vi "Private Read.vi"(8 "error in":errorcluster, 11 "Megger cluster in":T1={"Read data"={"Firmware version"="", "Model number"="", "Serial number"=0, "Ramp rate"=0.0, "Test Voltage"=0.0, "Test duration"=0.0, "Test stop watch"=0.0, "measured Current (nA)"=0.0, "calculated Resistance"=0.0, "Test Mode"=enum."Insulation resistance (IR)", "Test status"=enum."Waiting to start test"}, "Connected?"=FALSE, "Device status array"=[]}) -> (0 "error out":errorcluster, 2 "Serial read":string, 3 "Megger cluster out":T1={"Read data"={"Firmware version"="", "Model number"="", "Serial number"=0, "Ramp rate"=0.0, "Test Voltage"=0.0, "Test duration"=0.0, "Test stop watch"=0.0, "measured Current (nA)"=0.0, "calculated Resistance"=0.0, "Test Mode"=enum."Insulation resistance (IR)", "Test status"=enum."Waiting to start test"}, "Connected?"=FALSE, "Device status array"=[]})   [LabVIEW 2014]
uses:
  Controls/Megger cluster.ctl
  Controls/Global Megger.vi
  <vilib>/regexp/Match Regular Expression.xnode
  Stopwatch/Stop watch/Stop watch.lvlib
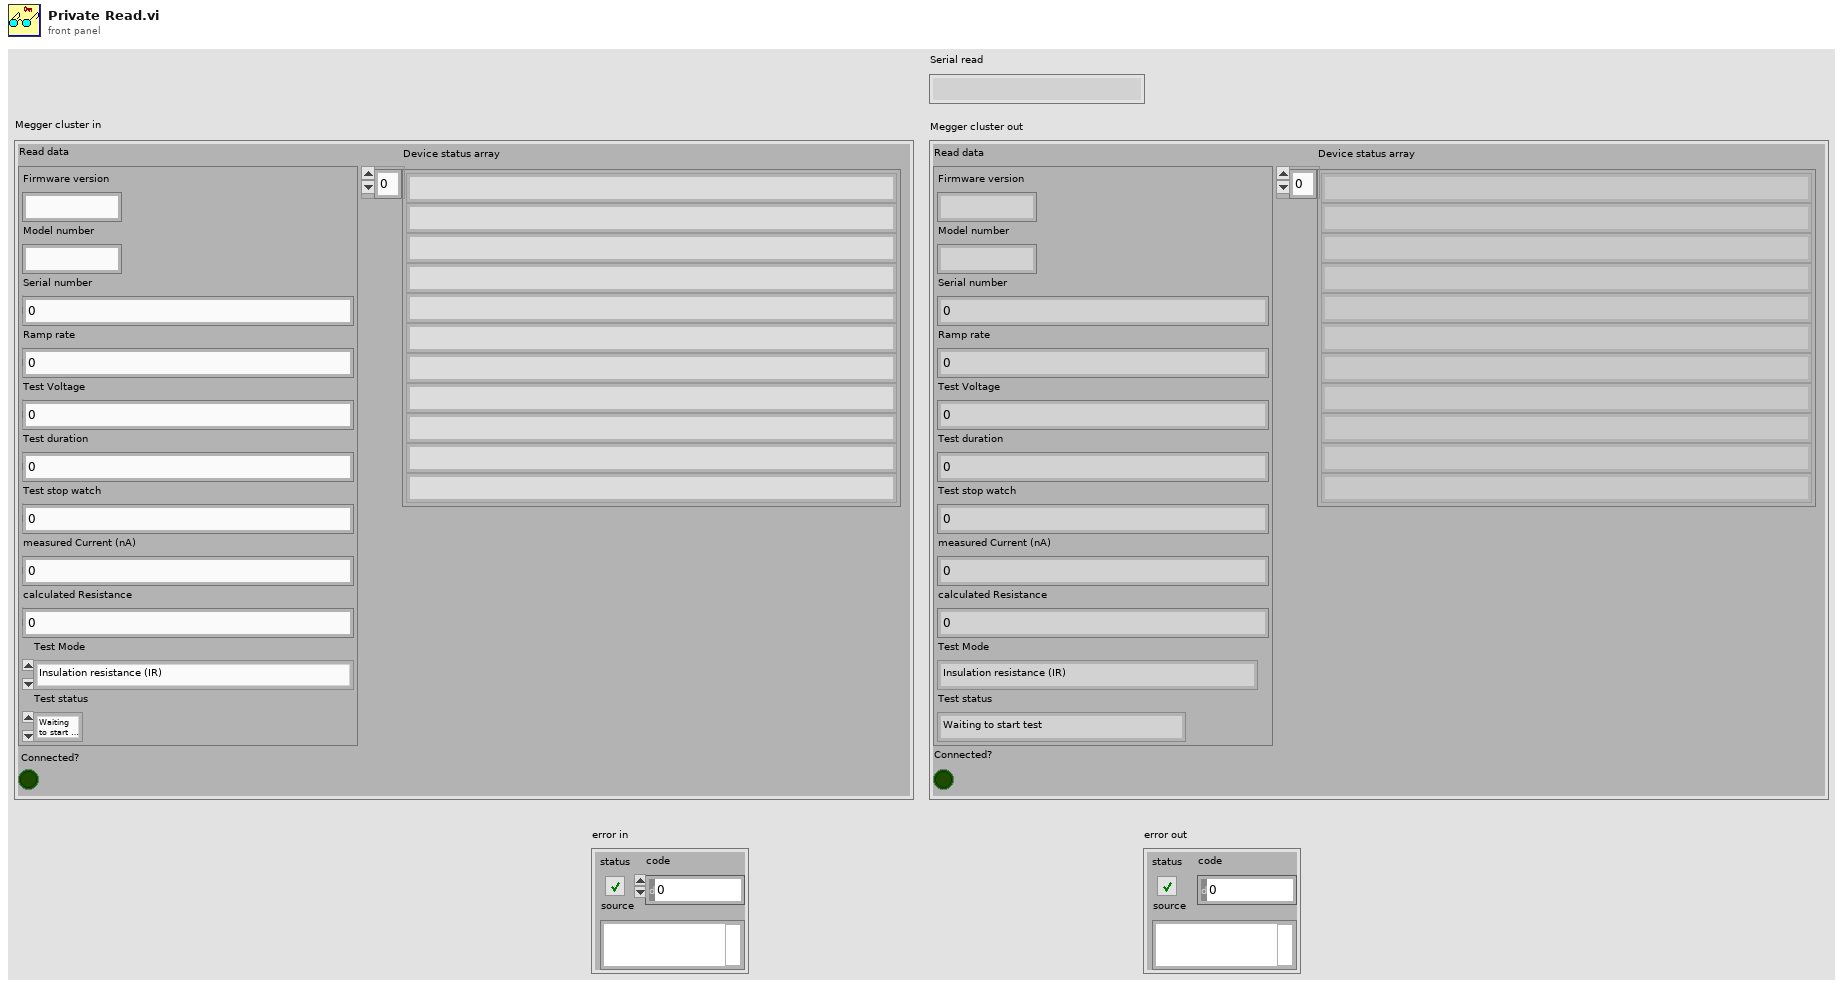
[diagram p1: front panel]
types:
  T1 = typedef "Megger cluster.ctl" = cluster{"Read data":cluster{"Firmware version":string, "Model number":string, "Serial number":i32, "Ramp rate":dbl, "Test Voltage":dbl, "Test duration":sgl, "Test stop watch":sgl, "measured Current (nA)":dbl, "calculated Resistance":dbl, "Test Mode":enum16{"N/A", "Insulation resistance (IR)", "Timed Insulation resistance (IR(t))", "Diaelectric Absorption Ratio (DAR)", "Polarisation Index (PI)", "Diaelectric Dishcharge (DD)", "Step voltage (SV)", "Ramp test (Ramp)"}, "Test status":enum16{"Waiting to start test", "Unable to start test", "Test progressing normally", "Performing post test measurements", "Test has ended normally", "Test has been aborted"}}, "Connected?":bool, "Device status array":string[]}
  T2 = enum16{"N/A", "Insulation resistance (IR)", "Timed Insulation resistance (IR(t))", "Diaelectric Absorption Ratio (DAR)", "Polarisation Index (PI)", "Diaelectric Dishcharge (DD)", "Step voltage (SV)", "Ramp test (Ramp)"}
  T3 = enum16{"Waiting to start test", "Unable to start test", "Test progressing normally", "Performing post test measurements", "Test has ended normally", "Test has been aborted"}
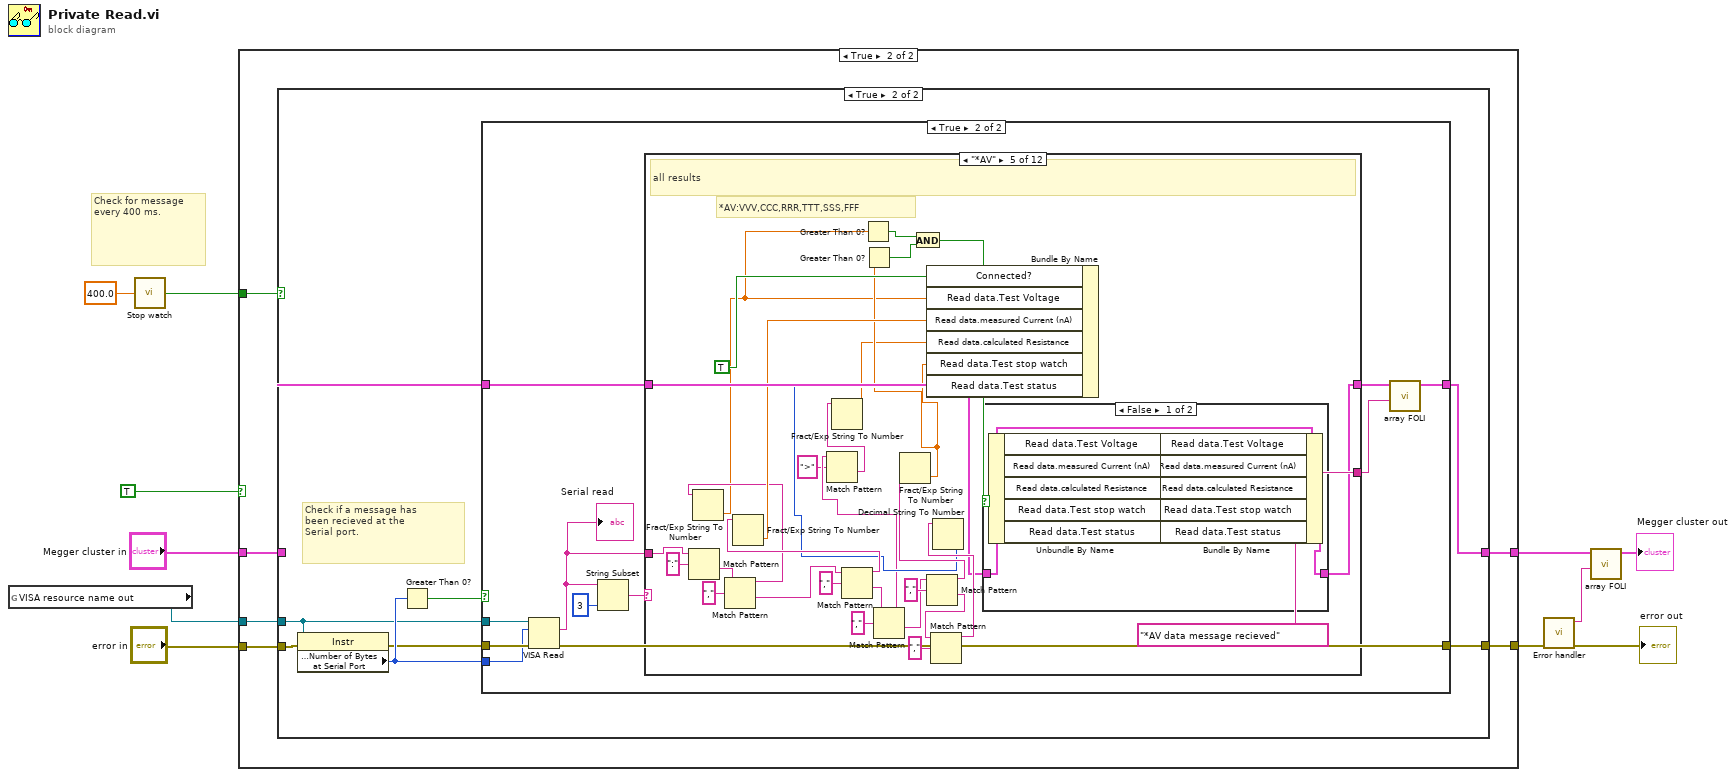
[diagram p0: block diagram]
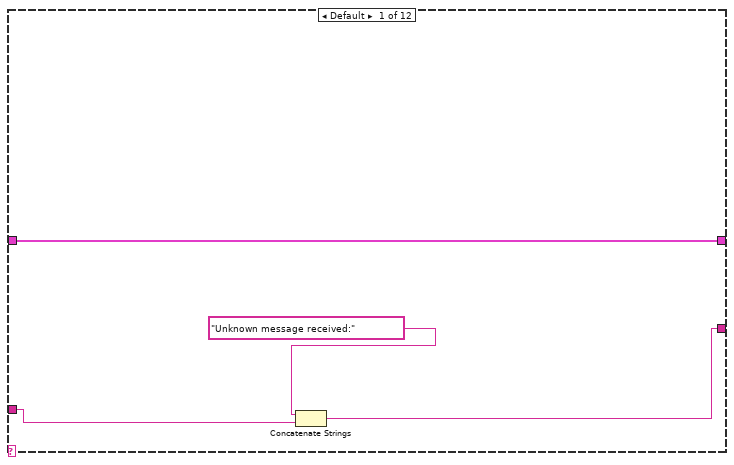
[diagram p5: hidden frame]
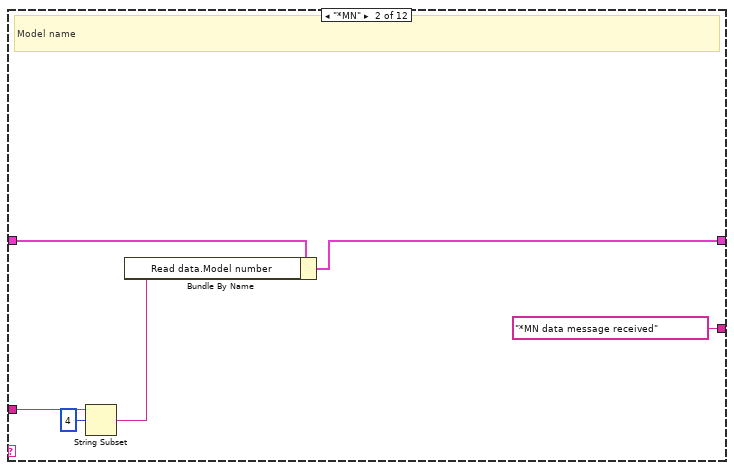
[diagram p6: hidden frame]
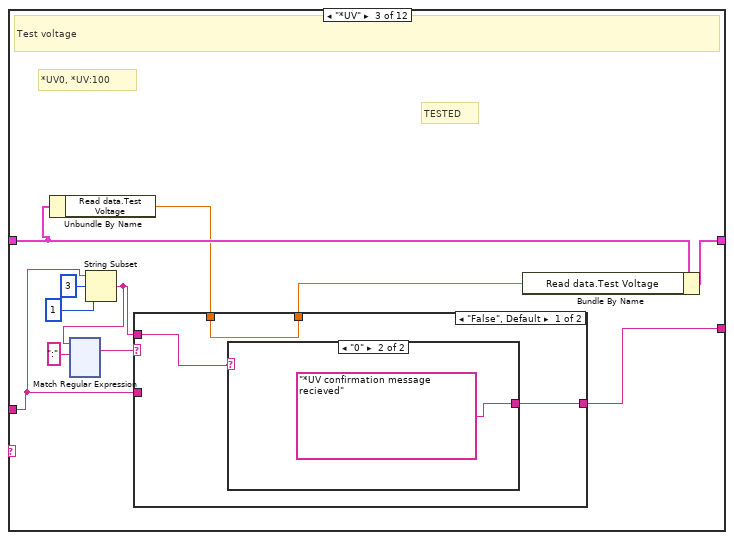
[diagram p7: hidden frame]
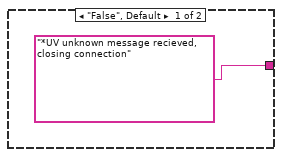
[diagram p8: hidden frame]
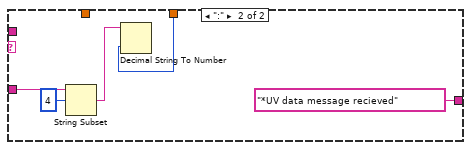
[diagram p9: hidden frame]
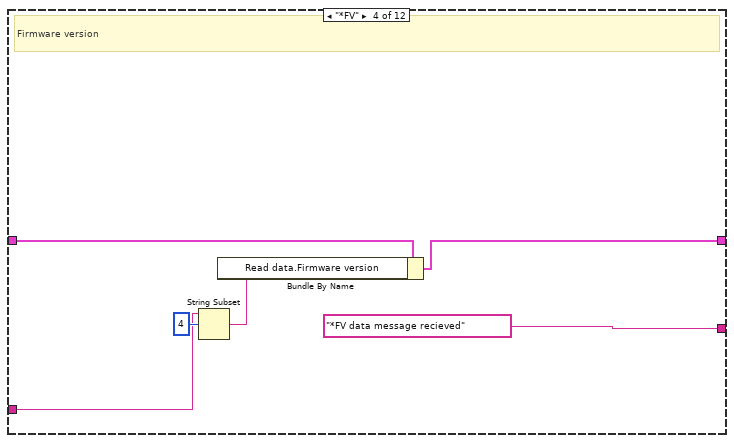
[diagram p10: hidden frame]
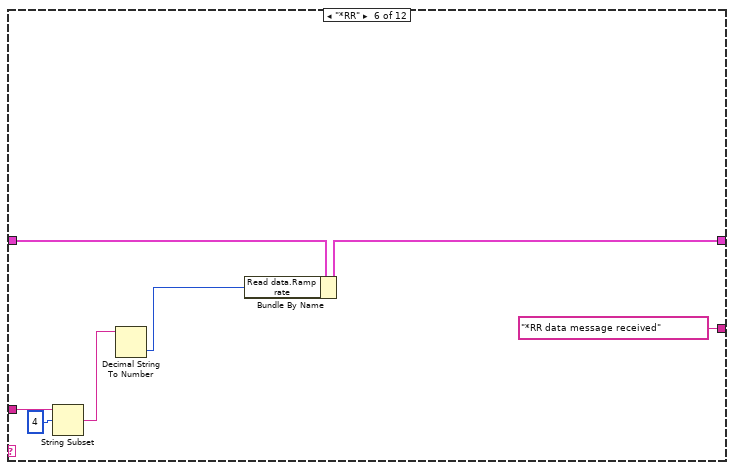
[diagram p12: hidden frame]
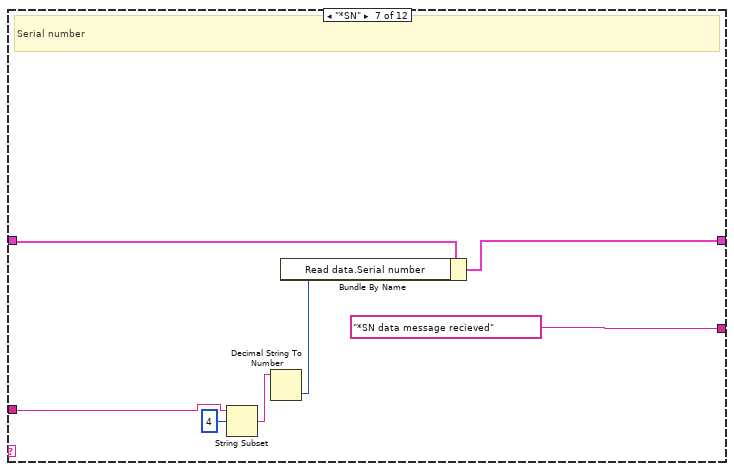
[diagram p13: hidden frame]
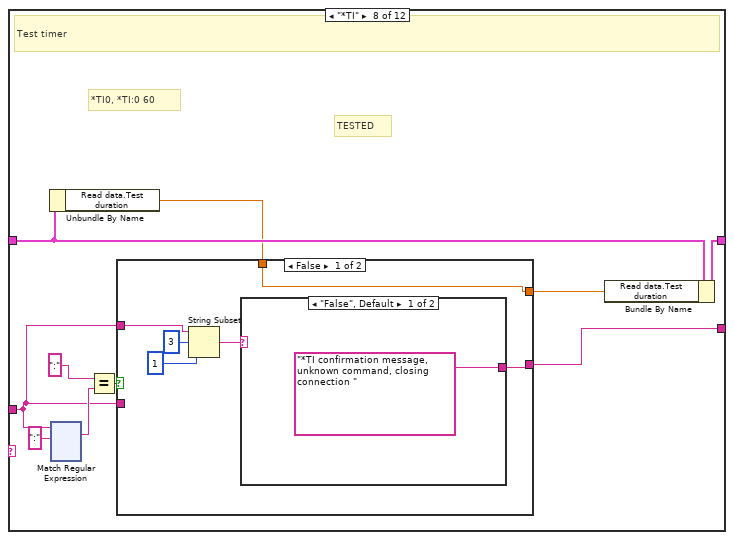
[diagram p14: hidden frame]
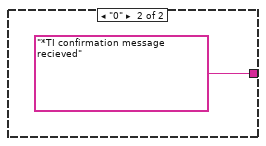
[diagram p15: hidden frame]
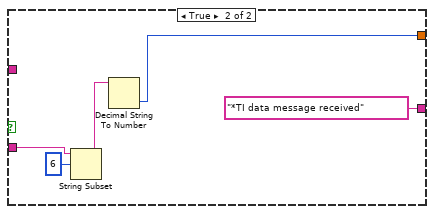
[diagram p16: hidden frame]
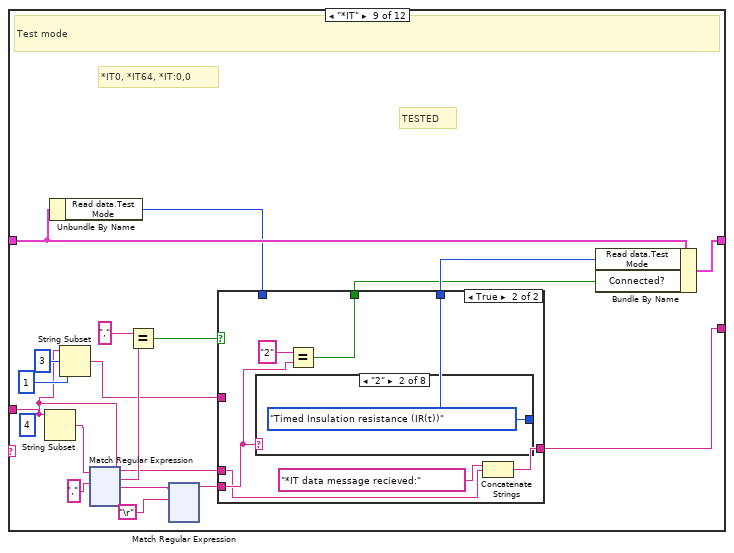
[diagram p17: hidden frame]
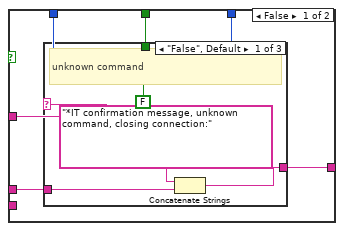
[diagram p18: hidden frame]
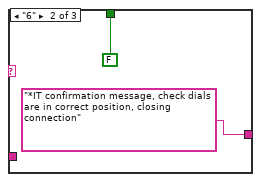
[diagram p19: hidden frame]
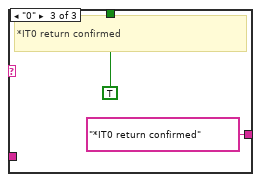
[diagram p20: hidden frame]
diagram:
  # "Check for message \nevery 400 ms."
  n1 = global read "Global Megger.vi" "VISA resource name out"() -> (w3:refnum<visa-resource-name>)
  n2 = call "Stop watch.vi"("Time to wait, mS"=400.0) -> ("Timer up"=w2:bool)  [unwired: 13 in, 1 out]
  n3 = case shown="True" TRUE {
    tunnel: [w13 w19] -> w8
    tunnel: "Megger cluster in" -> [w12 w18]
    tunnel: [w12 w17] -> w7
    tunnel: "error in" -> [w13 w16]
    tunnel: w2 -> [_ w15]
    tunnel: w3 -> [_ w14]
    frame False {
    }
    frame True {
      n4 = case shown="True" w15 {
        tunnel: [w21 w29] -> w19
        tunnel: w18 -> [w20 w28]
        tunnel: [w20 w27] -> w17
        tunnel: w16 -> [w21 w23]
        tunnel: w14 -> [_ w22]
        frame False {
        }
        frame True {
          # "Check if a message has \nbeen recieved at the\nSerial port."
          n5 = property class="Instr"(reference=w22, error in=w23) -> (error out=w24:errorcluster, "Serial Settings:Number of Bytes at Serial Port"=w25:u32)  [unwired: 1 out]
          n6 = Greater Than 0?(x=w25) -> (x > 0?=w26:bool)
          n7 = case shown="True" w26 {
            tunnel: [w31 w42] -> w29
            tunnel: w22 -> [_ w41]
            tunnel: w24 -> [w31 w40]
            tunnel: w25 -> [_ w39]
            tunnel: w28 -> [w30 w37]
            tunnel: [w30 w32] -> w27
            frame False {
            }
            frame True {
              n8 = VISA Read(VISA resource name=w41, byte count=w39, error in (no error)=w40) -> (read buffer=w36:string, error out=w42:errorcluster)  [unwired: 2 out]
              "Serial read" <- w36
              n9 = String Subset(string=w36, length (rest)=3 ("length (rest)")) -> (substring=w35:string)  [unwired: 1 in]
              n10 = case shown="\"*AV\"" w35 {
                tunnel: w36 -> [w45 w52 w58 w188 w220 w237 w244 w250 w388 w661 w668 w1063]
                tunnel: w37 -> [w46 w50 w54 w191 w219 w240 w243 w249 w390 w664 w666 w1060]
                tunnel: [w46 w49 w63 w190 w199 w239 w242 w257 w399 w663 w676 w1060] -> w34
                tunnel: [w43 "*MN data message received" ("x") w61 "*FV data message recieved" ("x") "*AV data message recieved" ("x") "*RR data message received" ("x") "*SN data message recieved" ("x") w251 w394 w659 w671 w1061] -> w33
                frame Default {
                  n11 = Concatenate Strings("Unknown message received:" ("x"), w45) -> (w43:string)
                }
                frame "*MN" {
                  # "Model name"
                  n12 = String Subset(string=w52, offset (0)=4) -> (substring=w48:string)  [unwired: 1 in]
                  n13 = Bundle By Name(cluster=w50, "Read data.Model number"=w48) -> (w49:T1)
                }
                frame "*UV" {
                  # "TESTED"
                  # "*UV0, *UV:100"
                  # "Test voltage"
                  n14 = Unbundle By Name(w54) -> ("Read data.Test Voltage"=w53:dbl)
                  n15 = String Subset(string=w58, offset (0)=3, length (rest)=1 ("length (rest)")) -> (substring=w55:string)
                  n16 = xnode "Match Regular Expression"("input string"=w55, "regular expression"=":") -> ("whole match"=w56:string)  [unwired: 4 in, 4 out]
                  n17 = case shown="\"False\", Default" w56 {
                    tunnel: [w64 w71] -> w62
                    tunnel: [w65 "*UV data message recieved"] -> w61
                    tunnel: w58 -> [_ w70]
                    tunnel: w55 -> [w66 _]
                    tunnel: w53 -> [w64 _]
                    frame "False", Default {
                      n18 = case shown="\"0\"" w66 {
                        tunnel: ["*UV unknown message recieved, closing connection" "*UV confirmation message recieved"] -> w65
                        frame "False", Default {
                        }
                        frame "0" {
                        }
                      }
                    }
                    frame ":" {
                      n19 = String Subset(string=w70, offset (0)=4) -> (substring=w72:string)  [unwired: 1 in]
                      n20 = Decimal String To Number(string=w72) -> (number=w71:i32)  [unwired: 2 in, 1 out]
                    }
                  }
                  n21 = Bundle By Name(cluster=w54, "Read data.Test Voltage"=w62) -> (w63:T1)
                }
                frame "*FV" {
                  # "Firmware version"
                  n22 = String Subset(string=w188, offset (0)=4) -> (substring=w193:string)  [unwired: 1 in]
                  n23 = Bundle By Name(cluster=w191, "Read data.Firmware version"=w193) -> (w190:T1)
                }
                frame "*AV" {
                  # "*AV:VVV,CCC,RRR,TTT,SSS,FFF"
                  # "all results"
                  n24 = Match Pattern(string=w220, regular expression=":") -> (after substring=w224:string)  [unwired: 1 in, 3 out]
                  n25 = Match Pattern(string=w224, regular expression=",") -> (before substring=w206:string, after substring=w221:string)  [unwired: 1 in, 2 out]
                  n26 = Fract/Exp String To Number(string=w206) -> (number=w203:dbl)  [unwired: 3 in, 1 out]
                  n27 = Match Pattern(string=w221, regular expression=",") -> (before substring=w218:string, after substring=w216:string)  [unwired: 1 in, 2 out]
                  n28 = Fract/Exp String To Number(string=w218) -> (number=w217:dbl)  [unwired: 3 in, 1 out]
                  n29 = Greater Than 0?(x=w203) -> (x > 0?=w202:bool)
                  n30 = Match Pattern(string=w216, regular expression=",") -> (before substring=w196:string, after substring=w212:string)  [unwired: 1 in, 2 out]
                  n31 = Match Pattern(string=w196, regular expression=">") -> (after substring=w194:string)  [unwired: 1 in, 3 out]
                  n32 = Fract/Exp String To Number(string=w194) -> (number=w197:dbl)  [unwired: 3 in, 1 out]
                  n33 = Match Pattern(string=w212, regular expression=",") -> (before substring=w213:string, after substring=w211:string)  [unwired: 1 in, 2 out]
                  n34 = Fract/Exp String To Number(string=w213) -> (number=w204:dbl)  [unwired: 3 in, 1 out]
                  n35 = Greater Than 0?(x=w204) -> (x > 0?=w201:bool)
                  n36 = And(x=w202, y=w201) -> (x .and. y?=w200:bool)
                  n37 = Match Pattern(string=w211, regular expression=",") -> (before substring=w209:string)  [unwired: 1 in, 3 out]
                  n38 = Decimal String To Number(string=w209) -> (number=w208:i32)  [unwired: 2 in, 1 out]
                  n39 = Bundle By Name(cluster=w219, "Connected?"=TRUE, "Read data.Test Voltage"=w203, "Read data.measured Current (nA)"=w217, "Read data.calculated Resistance"=w197, "Read data.Test stop watch"=w204, "Read data.Test status"=w208) -> (w198:T1)
                  n40 = case shown="False" w200 {
                    tunnel: [w226 w233] -> w199
                    tunnel: w198 -> [w227 w233]
                    frame False {
                      n41 = Unbundle By Name(w227) -> ("Read data.Test Voltage"=w228:dbl, "Read data.measured Current (nA)"=w229:dbl, "Read data.calculated Resistance"=w230:dbl, "Read data.Test stop watch"=w231:sgl, "Read data.Test status"=w232:T3)
                      n42 = Bundle By Name(cluster=w227, "Read data.Test Voltage"=w228, "Read data.measured Current (nA)"=w229, "Read data.calculated Resistance"=w230, "Read data.Test stop watch"=w231, "Read data.Test status"=w232) -> (w226:T1)
                    }
                    frame True {
                    }
                  }
                }
                frame "*RR" {
                  n43 = String Subset(string=w237, offset (0)=4) -> (substring=w236:string)  [unwired: 1 in]
                  n44 = Decimal String To Number(string=w236) -> (number=w235:i32)  [unwired: 2 in, 1 out]
                  n45 = Bundle By Name(cluster=w240, "Read data.Ramp rate"=w235) -> (w239:T1)
                }
                frame "*SN" {
                  # "Serial number"
                  n46 = String Subset(string=w244, offset (0)=4) -> (substring=w246:string)  [unwired: 1 in]
                  n47 = Decimal String To Number(string=w246) -> (number=w247:i32)  [unwired: 2 in, 1 out]
                  n48 = Bundle By Name(cluster=w243, "Read data.Serial number"=w247) -> (w242:T1)
                }
                frame "*TI" {
                  # "TESTED"
                  # "*TI0, *TI:0 60"
                  # "Test timer"
                  n49 = Unbundle By Name(w249) -> ("Read data.Test duration"=w248:sgl)
                  n50 = xnode "Match Regular Expression"("input string"=w250, "regular expression"=":") -> ("whole match"=w253:string)  [unwired: 4 in, 4 out]
                  n51 = Equal?(x=":" ("regular expression"), y=w253) -> (x = y?=w252:bool)
                  n52 = case shown="False" w252 {
                    tunnel: [w258 w268] -> w256
                    tunnel: w250 -> [_ w267]
                    tunnel: [w259 "*TI data message received" ("x")] -> w251
                    tunnel: w250 -> [w261 _]
                    tunnel: w248 -> [w258 _]
                    frame False {
                      n53 = String Subset(string=w261, offset (0)=3, length (rest)=1 ("length (rest)")) -> (substring=w260:string)
                      n54 = case shown="\"False\", Default" w260 {
                        tunnel: ["*TI confirmation message, unknown command, closing connection " ("x") "*TI confirmation message recieved" ("x")] -> w259
                        frame "False", Default {
                        }
                        frame "0" {
                        }
                      }
                    }
                    frame True {
                      n55 = String Subset(string=w267, offset (0)=6) -> (substring=w269:string)  [unwired: 1 in]
                      n56 = Decimal String To Number(string=w269) -> (number=w268:i32)  [unwired: 2 in, 1 out]
                    }
                  }
                  n57 = Bundle By Name(cluster=w249, "Read data.Test duration"=w256) -> (w257:T1)
                }
                frame "*IT" {
                  (unwired) 4 ("offset (0)")
                  # "TESTED"
                  # "*IT0, *IT64, *IT:0,0"
                  # "Test mode"
                  n58 = String Subset(string=w388) -> (substring=w401:string)  [unwired: 2 in]
                  n59 = Unbundle By Name(w390) -> ("Read data.Test Mode"=w389:T2)
                  n60 = String Subset(string=w388, offset (0)=3, length (rest)=1 ("length (rest)")) -> (substring=w391:string)
                  n61 = xnode "Match Regular Expression"("input string"=w401, "regular expression"=",") -> ("whole match"=w396:string, "after match"=w386:string)  [unwired: 4 in, 3 out]
                  n62 = Equal?(x=",", y=w396) -> (x = y?=w395:bool)
                  n63 = xnode "Match Regular Expression"("input string"=w386, "regular expression"="\r") -> ("before match"=w385:string)  [unwired: 4 in, 4 out]
                  n64 = case shown="True" w395 {
                    tunnel: [w518 w536] -> w400
                    tunnel: [w521 w534] -> w398
                    tunnel: w391 -> [w519 _]
                    tunnel: [w520 w532] -> w394
                    tunnel: w389 -> [w518 _]
                    tunnel: w388 -> [w517 w530]
                    tunnel: w385 -> [_ w531]
                    frame False {
                      n65 = case shown="\"False\", Default" w519 {
                        tunnel: [FALSE FALSE TRUE] -> w521
                        tunnel: [w523 "*IT confirmation message, check dials are in correct position, closing connection" ("x") "*IT0 return confirmed" ("x")] -> w520
                        tunnel: w517 -> [w522 _ _]
                        frame "False", Default {
                          # "unknown command"
                          n66 = Concatenate Strings("*IT confirmation message, unknown command, closing connection:" ("x"), w522) -> (w523:string)
                        }
                        frame "6" {
                        }
                        frame "0" {
                          # "*IT0 return confirmed"
                        }
                      }
                    }
                    frame True {
                      n67 = case shown="\"2\"" w531 {
                        tunnel: [T2."Insulation resistance (IR)" T2."Timed Insulation resistance (IR(t))" T2."Diaelectric Absorption Ratio (DAR)" T2."Polarisation Index (PI)" T2."Diaelectric Dishcharge (DD)" T2."Step voltage (SV)" T2."Ramp test (Ramp)" T2."N/A"] -> w536
                        frame "1" {
                        }
                        frame "2" {
                        }
                        frame "3" {
                        }
                        frame "4" {
                        }
                        frame "5" {
                        }
                        frame "6" {
                        }
                        frame "7" {
                        }
                        frame "0", Default {
                        }
                      }
                      n68 = Equal?(x="2", y=w531) -> (x = y?=w534:bool)
                      n69 = Concatenate Strings("*IT data message recieved:" ("x"), w530) -> (w532:string)
                    }
                  }
                  n70 = Bundle By Name(cluster=w390, "Read data.Test Mode"=w400, "Connected?"=w398) -> (w399:T1)
                }
                frame "*ER" {
                  # "error code"
                  n71 = Bundle By Name(cluster=w664, "Connected?"=FALSE) -> (w663:T1)
                  n72 = Concatenate Strings("*ER error message received, closing connection:" ("x"), w661) -> (w659:string)
                }
                frame "*TS" {
                  # "*TS0"
                  # "*TS:0,0,0"
                  # "1. test status, 0 = waiting to start test \n2. flag bits sent in a byte, 0 no error\n3. error code"
                  # "test status"
                  n73 = Unbundle By Name(w666) -> ("Read data.Test status"=w665:T3)
                  n74 = String Subset(string=w668, offset (0)=4) -> (substring=w682:string)  [unwired: 1 in]
                  n75 = String Subset(string=w668, offset (0)=3, length (rest)=1 ("length (rest)")) -> (substring=w667:string)
                  n76 = xnode "Match Regular Expression"("input string"=w682, "regular expression"=",") -> ("before match"=w678:string, "whole match"=w674:string, "after match"=w679:string)  [unwired: 4 in, 2 out]
                  n77 = Equal?(x="," ("regular expression"), y=w674) -> (x = y?=w672:bool)
                  n78 = case shown="True" w672 {
                    tunnel: w679 -> [_ w704]
                    tunnel: w678 -> [_ w700]
                    tunnel: [w683 w699] -> w677
                    tunnel: [w684 w698] -> w675
                    tunnel: [w685 w694] -> w671
                    tunnel: w667 -> [w686 _]
                    tunnel: w665 -> [w683 _]
                    frame False {
                      n79 = case shown="\"False\", Default" w686 {
                        tunnel: ["*TS confirmation message recieved, unknown command, closing connection" ("x") "*TS confirmation message recieved" ("x")] -> w685
                        tunnel: [FALSE TRUE] -> w684
                        frame "False", Default {
                        }
                        frame "0" {
                        }
                      }
                    }
                    frame True {
                      n80 = Decimal String To Number(string=w700) -> (number=w699:i32)  [unwired: 2 in, 1 out]
                      n81 = xnode "Match Regular Expression"("input string"=w704, "regular expression"=",") -> ("before match"=w703:string, "after match"=w693:string)  [unwired: 4 in, 3 out]
                      n82 = case shown="\"1\", Default" w703 {
                        selector: w703 -> [w828 _]
                        tunnel: [FALSE TRUE] -> w701
                        tunnel: [w826 ""] -> w696
                        frame "1", Default {
                          n83 = Concatenate Strings(", flag bit error:", w828) -> (w826:string)
                        }
                        frame "0" {
                        }
                      }
                      n84 = xnode "Match Regular Expression"("input string"=w693, "regular expression"="\r") -> ("before match"=w691:string)  [unwired: 4 in, 4 out]
                      n85 = case shown="\"1\", Default" w691 {
                        selector: w691 -> [w821 _]
                        tunnel: [FALSE TRUE] -> w702
                        tunnel: [w820 ""] -> w697
                        frame "1", Default {
                          n86 = Concatenate Strings(", fatal error:" ("x"), w821) -> (w820:string)
                        }
                        frame "0" {
                        }
                      }
                      n87 = Concatenate Strings("*TS data message recieved" ("x"), w696, w697) -> (w694:string)
                      n88 = And(x=w701, y=w702) -> (x .and. y?=w698:bool)
                    }
                  }
                  n89 = Bundle By Name(cluster=w666, "Connected?"=w675, "Read data.Test status"=w677) -> (w676:T1)
                }
                frame "*ST" {
                  # "*ST0"
                  # "Start test"
                  n90 = String Subset(string=w1063, offset (0)=3, length (rest)=1 ("length (rest)")) -> (substring=w1062:string)
                  n91 = case shown="\"False\", Default" w1062 {
                    tunnel: ["*ST unknown message recieved" "*ST0 confirmation message. Test started."] -> w1061
                    frame "False", Default {
                    }
                    frame "0" {
                    }
                  }
                }
              }
              n92 = call "array FOLI.vi"("status string"=w33, "Megger cluster in"=w34) -> ("Megger cluster out"=w32:T1)  [unwired: 9 in]
            }
          }
        }
      }
    }
  }
  n93 = call "Error handler.vi"("error in"=w8) -> ("error out"=→"error out":errorcluster, "Status string"=w6:string)  [unwired: 8 in, 1 out]
  n94 = call "array FOLI.vi"("status string"=w6, "Megger cluster in"=w7) -> ("Megger cluster out"=→"Megger cluster out":T1)  [unwired: 9 in]
